vi "Profile_Read.vi"(7 "Measurement Profile":path, 8 "error in (no error)":errorcluster, 10 "Configuration Cluster":T1={"General"={"Config.ini"=path "", "Default Logging Path"=path ""}, "Hardware"={"LCR VISA COM"="", "Measure Rate (1/s)"=0, "Reset on Load?"=FALSE, "Measure Profile"=path ""}, "HM8118 Current Profile"={"Bias Profile"={" Bias Source (OFF)"=0, " Bias Type (Voltage)"=0, "Bias Level (0)"=0.0}, "Measurement Profile"={"Operation Mode (0: Auto)"=0, "Circuit Type (2: Auto)"=2, "Manual Range (1:Range 1 and 25 Ohms)"=1, "Auto Range (T: Enable)"=TRUE}, "Signal Profile"={"Frequency (1kHz)"=1000.0, "Measuring Voltage (1V)"=1.0}, "Integration Profile"={"Averaging (0: Off)"=0, "Averaging Number (2)"=2, "Time (100ms)"=100, "Rate (0: Fast)"=0}, "Trigger Profile"={"Trigger Mode (0: Continuous)"=0}}, "HM8118 New Profile"={"Bias Profile"={" Bias Source (OFF)"=0, " Bias Type (Voltage)"=0, "Bias Level (0)"=0.0}, "Measurement Profile"={"Operation Mode (0: Auto)"=0, "Circuit Type (2: Auto)"=2, "Manual Range (1:Range 1 and 25 Ohms)"=1, "Auto Range (T: Enable)"=TRUE}, "Signal Profile"={"Frequency (1kHz)"=1000.0, "Measuring Voltage (1V)"=1.0}, "Integration Profile"={"Averaging (0: Off)"=0, "Averaging Number (2)"=2, "Time (100ms)"=100, "Rate (0: Fast)"=0}, "Trigger Profile"={"Trigger Mode (0: Continuous)"=0}}, "Operation"={"Operation Mode"=enum."Logging", "Status"=""}} {"HM8118 New Profile"."Trigger Profile"."Trigger Mode (0: Continuous)" items=["Continuous", "Manual", "External"]; "HM8118 New Profile"."Integration Profile"."Rate (0: Fast)" items=["Fast", "Medium", "Slow"]; "HM8118 New Profile"."Integration Profile"."Time (100ms)" min=1 max=999; "HM8118 New Profile"."Integration Profile"."Averaging Number (2)" min=2 max=99; "HM8118 New Profile"."Integration Profile"."Averaging (0: Off)" items=["Off", "Normal", "Averaging"]; "HM8118 New Profile"."Signal Profile"."Measuring Voltage (1V)" min=0.05 max=1.5 step=0.01; "HM8118 New Profile"."Signal Profile"."Frequency (1kHz)" min=20.0 max=200000.0; "HM8118 New Profile"."Measurement Profile"."Manual Range (1:Range 1 and 25 Ohms)" items=["Range 1 and 25 Ohms"=1, "Range 2 and 25 Ohms"=2, "Range 3 and 400 Ohms"=3, "Range 4 and 6.4 kOhms"=4, "Range 5 and 100kOhms"=5, "Range 6 and 100kOhms"=6]; "HM8118 New Profile"."Measurement Profile"."Circuit Type (2: Auto)" items=["Series", "Parallel", "Auto"]; "HM8118 New Profile"."Measurement Profile"."Operation Mode (0: Auto)" items=["Auto", "L+Q", "L+R", "C+D", "C+R", "R+Q", "Z+Theta", "Y+Theta", "R+X", "G+B", "N+Theta", "M"]; "HM8118 New Profile"."Bias Profile"."Bias Type (Voltage)" items=["Voltage", "Current"]; "HM8118 New Profile"."Bias Profile"."Bias Source (OFF)" items=["Off", "Internal", "External"]; "HM8118 Current Profile"."Trigger Profile"."Trigger Mode (0: Continuous)" items=["Continuous", "Manual", "External"]; "HM8118 Current Profile"."Integration Profile"."Rate (0: Fast)" items=["Fast", "Medium", "Slow"]; "HM8118 Current Profile"."Integration Profile"."Time (100ms)" min=1 max=999; "HM8118 Current Profile"."Integration Profile"."Averaging Number (2)" min=2 max=99; "HM8118 Current Profile"."Integration Profile"."Averaging (0: Off)" items=["Off", "Normal", "Averaging"]; "HM8118 Current Profile"."Signal Profile"."Measuring Voltage (1V)" min=0.05 max=1.5 step=0.01; "HM8118 Current Profile"."Signal Profile"."Frequency (1kHz)" min=20.0 max=200000.0; "HM8118 Current Profile"."Measurement Profile"."Manual Range (1:Range 1 and 25 Ohms)" items=["Range 1 and 25 Ohms"=1, "Range 2 and 25 Ohms"=2, "Range 3 and 400 Ohms"=3, "Range 4 and 6.4 kOhms"=4, "Range 5 and 100kOhms"=5, "Range 6 and 100kOhms"=6]; "HM8118 Current Profile"."Measurement Profile"."Circuit Type (2: Auto)" items=["Series", "Parallel", "Auto"]; "HM8118 Current Profile"."Measurement Profile"."Operation Mode (0: Auto)" items=["Auto", "L+Q", "L+R", "C+D", "C+R", "R+Q", "Z+Theta", "Y+Theta", "R+X", "G+B", "N+Theta", "M"]; "HM8118 Current Profile"."Bias Profile"."Bias Type (Voltage)" items=["Voltage", "Current"]; "HM8118 Current Profile"."Bias Profile"."Bias Source (OFF)" items=["Off", "Internal", "External"]}) -> (0 "error out":errorcluster, 2 "Configuration Cluster Out":T1={"General"={"Config.ini"=path "", "Default Logging Path"=path ""}, "Hardware"={"LCR VISA COM"="", "Measure Rate (1/s)"=0, "Reset on Load?"=FALSE, "Measure Profile"=path ""}, "HM8118 Current Profile"={"Bias Profile"={" Bias Source (OFF)"=0, " Bias Type (Voltage)"=0, "Bias Level (0)"=0.0}, "Measurement Profile"={"Operation Mode (0: Auto)"=0, "Circuit Type (2: Auto)"=2, "Manual Range (1:Range 1 and 25 Ohms)"=1, "Auto Range (T: Enable)"=TRUE}, "Signal Profile"={"Frequency (1kHz)"=1000.0, "Measuring Voltage (1V)"=1.0}, "Integration Profile"={"Averaging (0: Off)"=0, "Averaging Number (2)"=2, "Time (100ms)"=100, "Rate (0: Fast)"=0}, "Trigger Profile"={"Trigger Mode (0: Continuous)"=0}}, "HM8118 New Profile"={"Bias Profile"={" Bias Source (OFF)"=0, " Bias Type (Voltage)"=0, "Bias Level (0)"=0.0}, "Measurement Profile"={"Operation Mode (0: Auto)"=0, "Circuit Type (2: Auto)"=2, "Manual Range (1:Range 1 and 25 Ohms)"=1, "Auto Range (T: Enable)"=TRUE}, "Signal Profile"={"Frequency (1kHz)"=1000.0, "Measuring Voltage (1V)"=1.0}, "Integration Profile"={"Averaging (0: Off)"=0, "Averaging Number (2)"=2, "Time (100ms)"=100, "Rate (0: Fast)"=0}, "Trigger Profile"={"Trigger Mode (0: Continuous)"=0}}, "Operation"={"Operation Mode"=enum."Logging", "Status"=""}} {"HM8118 New Profile"."Trigger Profile"."Trigger Mode (0: Continuous)" items=["Continuous", "Manual", "External"]; "HM8118 New Profile"."Integration Profile"."Rate (0: Fast)" items=["Fast", "Medium", "Slow"]; "HM8118 New Profile"."Integration Profile"."Time (100ms)" min=1 max=999; "HM8118 New Profile"."Integration Profile"."Averaging Number (2)" min=2 max=99; "HM8118 New Profile"."Integration Profile"."Averaging (0: Off)" items=["Off", "Normal", "Averaging"]; "HM8118 New Profile"."Signal Profile"."Measuring Voltage (1V)" min=0.05 max=1.5 step=0.01; "HM8118 New Profile"."Signal Profile"."Frequency (1kHz)" min=20.0 max=200000.0; "HM8118 New Profile"."Measurement Profile"."Manual Range (1:Range 1 and 25 Ohms)" items=["Range 1 and 25 Ohms"=1, "Range 2 and 25 Ohms"=2, "Range 3 and 400 Ohms"=3, "Range 4 and 6.4 kOhms"=4, "Range 5 and 100kOhms"=5, "Range 6 and 100kOhms"=6]; "HM8118 New Profile"."Measurement Profile"."Circuit Type (2: Auto)" items=["Series", "Parallel", "Auto"]; "HM8118 New Profile"."Measurement Profile"."Operation Mode (0: Auto)" items=["Auto", "L+Q", "L+R", "C+D", "C+R", "R+Q", "Z+Theta", "Y+Theta", "R+X", "G+B", "N+Theta", "M"]; "HM8118 New Profile"."Bias Profile"."Bias Type (Voltage)" items=["Voltage", "Current"]; "HM8118 New Profile"."Bias Profile"."Bias Source (OFF)" items=["Off", "Internal", "External"]; "HM8118 Current Profile"."Trigger Profile"."Trigger Mode (0: Continuous)" items=["Continuous", "Manual", "External"]; "HM8118 Current Profile"."Integration Profile"."Rate (0: Fast)" items=["Fast", "Medium", "Slow"]; "HM8118 Current Profile"."Integration Profile"."Time (100ms)" min=1 max=999; "HM8118 Current Profile"."Integration Profile"."Averaging Number (2)" min=2 max=99; "HM8118 Current Profile"."Integration Profile"."Averaging (0: Off)" items=["Off", "Normal", "Averaging"]; "HM8118 Current Profile"."Signal Profile"."Measuring Voltage (1V)" min=0.05 max=1.5 step=0.01; "HM8118 Current Profile"."Signal Profile"."Frequency (1kHz)" min=20.0 max=200000.0; "HM8118 Current Profile"."Measurement Profile"."Manual Range (1:Range 1 and 25 Ohms)" items=["Range 1 and 25 Ohms"=1, "Range 2 and 25 Ohms"=2, "Range 3 and 400 Ohms"=3, "Range 4 and 6.4 kOhms"=4, "Range 5 and 100kOhms"=5, "Range 6 and 100kOhms"=6]; "HM8118 Current Profile"."Measurement Profile"."Circuit Type (2: Auto)" items=["Series", "Parallel", "Auto"]; "HM8118 Current Profile"."Measurement Profile"."Operation Mode (0: Auto)" items=["Auto", "L+Q", "L+R", "C+D", "C+R", "R+Q", "Z+Theta", "Y+Theta", "R+X", "G+B", "N+Theta", "M"]; "HM8118 Current Profile"."Bias Profile"."Bias Type (Voltage)" items=["Voltage", "Current"]; "HM8118 Current Profile"."Bias Profile"."Bias Source (OFF)" items=["Off", "Internal", "External"]})   [LabVIEW 2021]
uses:
  Config_Cluster.ctl
  Mode_Enum.ctl
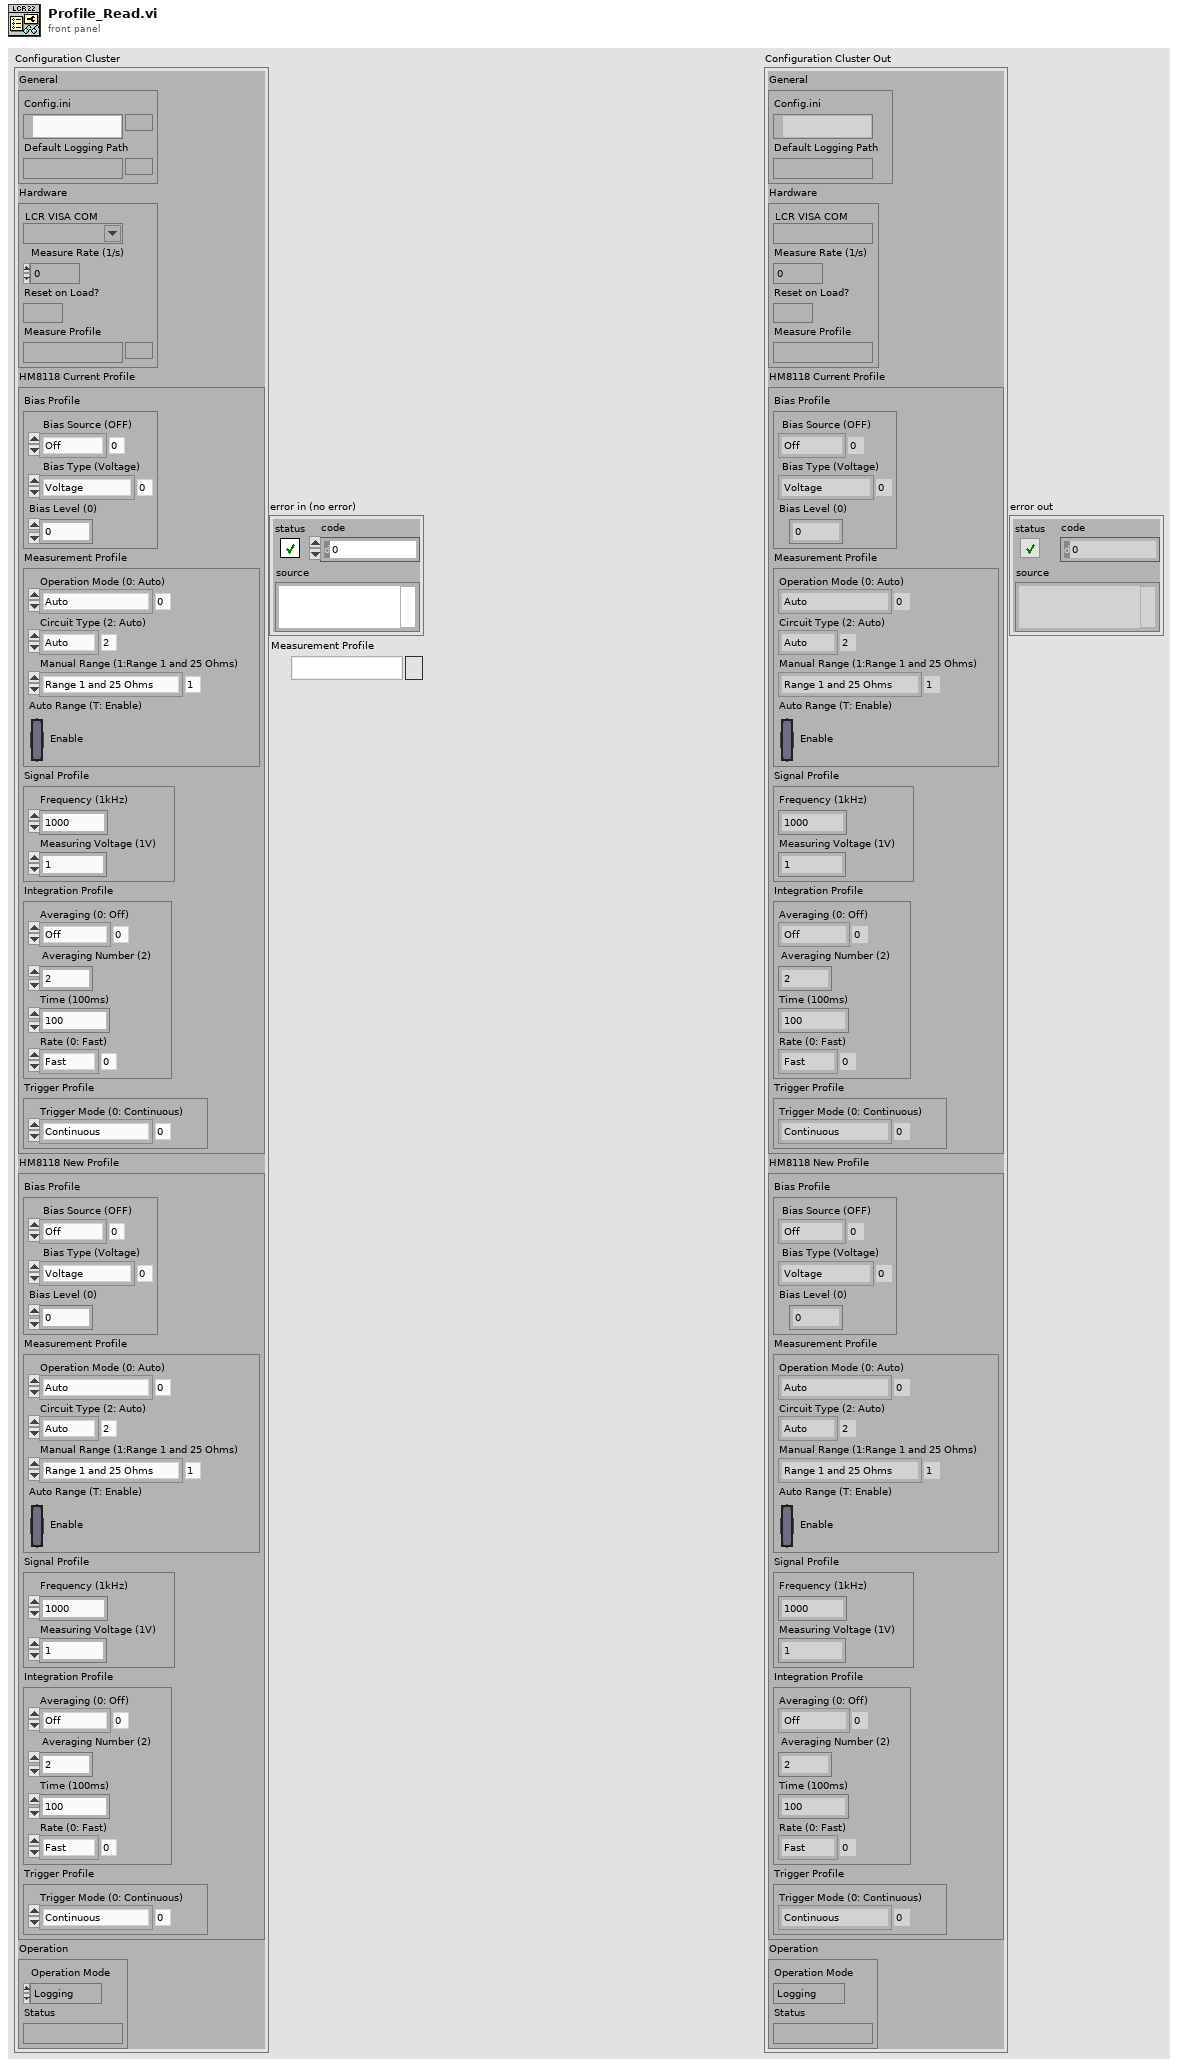
[diagram p1: front panel]
types:
  T1 = typedef "Config_Cluster.ctl" = cluster{"General":cluster{"Config.ini":path, "Default Logging Path":path}, "Hardware":cluster{"LCR VISA COM":refnum<visa-resource-name>, "Measure Rate (1/s)":i32, "Reset on Load?":bool, "Measure Profile":path}, "HM8118 Current Profile":cluster{"Bias Profile":cluster{" Bias Source (OFF)":u8, " Bias Type (Voltage)":u8, "Bias Level (0)":dbl}, "Measurement Profile":cluster{"Operation Mode (0: Auto)":u16, "Circuit Type (2: Auto)":u16, "Manual Range (1:Range 1 and 25 Ohms)":u8, "Auto Range (T: Enable)":bool}, "Signal Profile":cluster{"Frequency (1kHz)":dbl, "Measuring Voltage (1V)":dbl}, "Integration Profile":cluster{"Averaging (0: Off)":u16, "Averaging Number (2)":i32, "Time (100ms)":i32, "Rate (0: Fast)":u16}, "Trigger Profile":cluster{"Trigger Mode (0: Continuous)":u16}}, "HM8118 New Profile":cluster{"Bias Profile":cluster{" Bias Source (OFF)":u8, " Bias Type (Voltage)":u8, "Bias Level (0)":dbl}, "Measurement Profile":cluster{"Operation Mode (0: Auto)":u16, "Circuit Type (2: Auto)":u16, "Manual Range (1:Range 1 and 25 Ohms)":u8, "Auto Range (T: Enable)":bool}, "Signal Profile":cluster{"Frequency (1kHz)":dbl, "Measuring Voltage (1V)":dbl}, "Integration Profile":cluster{"Averaging (0: Off)":u16, "Averaging Number (2)":i32, "Time (100ms)":i32, "Rate (0: Fast)":u16}, "Trigger Profile":cluster{"Trigger Mode (0: Continuous)":u16}}, "Operation":cluster{"Operation Mode":T2, "Status":string}}
  T2 = typedef "Mode_Enum.ctl" = enum16{"Logging", "Idle-Off", "Idle"}
  T3 = cluster{"Bias Profile":cluster{" Bias Source (OFF)":u8, " Bias Type (Voltage)":u8, "Bias Level (0)":dbl}, "Measurement Profile":cluster{"Operation Mode (0: Auto)":u16, "Circuit Type (2: Auto)":u16, "Manual Range (1:Range 1 and 25 Ohms)":u8, "Auto Range (T: Enable)":bool}, "Signal Profile":cluster{"Frequency (1kHz)":dbl, "Measuring Voltage (1V)":dbl}, "Integration Profile":cluster{"Averaging (0: Off)":u16, "Averaging Number (2)":i32, "Time (100ms)":i32, "Rate (0: Fast)":u16}, "Trigger Profile":cluster{"Trigger Mode (0: Continuous)":u16}}
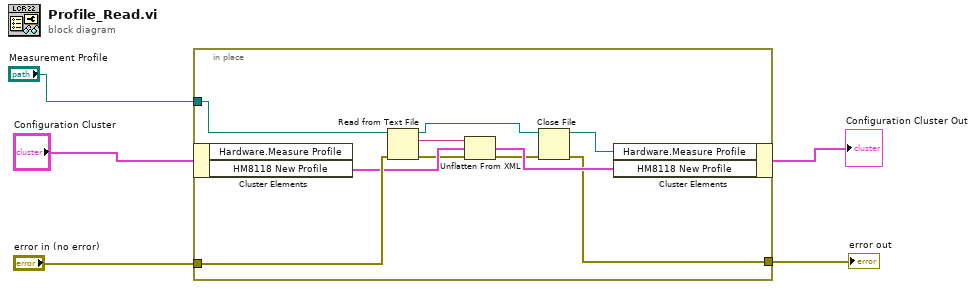
[diagram p0: block diagram]
diagram:
  n1 = in-place {
    in-place-border: "Measurement Profile" -> [w15]
    in-place-border: "error in (no error)" -> [w14]
    in-place-border: [w7] -> w1
    n2 = in-place-cluster #1("Configuration Cluster") -> ("HM8118 New Profile"=w12:T3)  [unwired: 1 out]
    n3 = Read from Text File(file (use dialog)=w15, error in=w14) -> (refnum out=w9:refnum<file>, text=w13:string, error out=w11:errorcluster)  [unwired: 2 in, 1 out]
    n4 = Unflatten From XML(xml string=w13, type=w12, error in (no error)=w11) -> (value=w10:T3, error out=w8:errorcluster)
    n5 = Close File(refnum=w9, error in=w8) -> (path=w6:path, error out=w7:errorcluster)
    n6 = in-place-cluster #1("Hardware.Measure Profile"=w6, "HM8118 New Profile"=w10) -> (→"Configuration Cluster Out":T1)
  }
  "error out" <- w1
